vi "Hash ID.vi"(11 "ID":string) -> (3 "Hashed ID":string)   [LabVIEW 2020, in "HTTP Server.lvlib" / "Session.lvclass"]
uses:
  Session.lvclass
  lv-web-crypto/lv-base64/Variant.ctl
  lv-web-crypto/lv-crypto/Crypto/Hashes/SHA-256/SHA-256.lvclass
  lv-web-crypto/lv-base64/Base64.lvlib
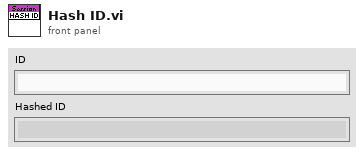
[diagram p1: front panel]
types:
  T1 = typedef "Base64.lvlib/Variant.ctl" = enum16{"Base64", "Base64-URL"}
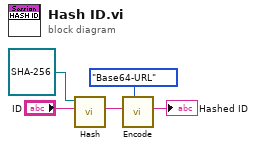
[diagram p0: block diagram]
diagram:
  n1 = call-dynamic "Hash.vi"("Message"="ID", "SHA-256 in"=refnum<class "SHA-256.lvclass"> refnum ("Crypto.lvlib:SHA-256.lvclass")) -> ("Hash"=w4:string)  [unwired: 7 in, 2 out]
  n2 = call "Encode.vi"("Variant (Base64)"=Variant."Base64-URL", "string in (not encoded)"=w4) -> ("string out (base64-encoded)"=→"Hashed ID":string)  [unwired: 8 in, 1 out]
